vi "點檢_VI_畫十字線.vi"(8 "error in (no error)":errorcluster, 11 "Refnum in":T1) -> (0 "error out":errorcluster, 2 "中心點":cluster{sgl, sgl}, 3 "Refnum out":T1)   [LabVIEW 2015]
uses:
  <vilib>/vision/Image Controls.llb/IMAQ Image.ctl
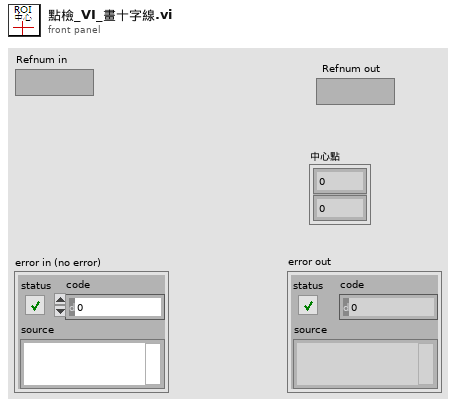
[diagram p1: front panel]
types:
  T1 = typedef "IMAQ Image.ctl" = refnum<image>
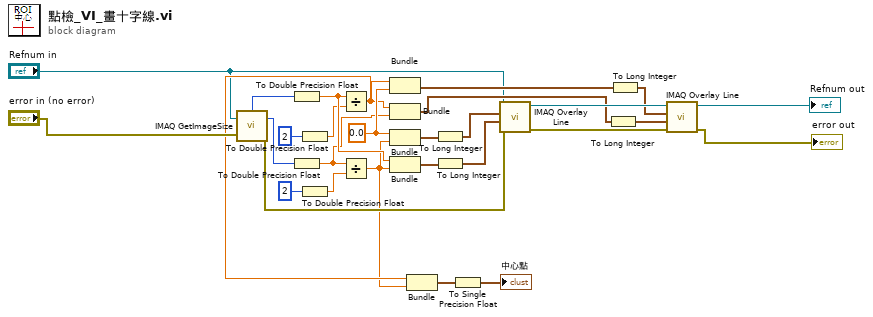
[diagram p0: block diagram]
diagram:
  w20 = 0.0
  n1 = call "IMAQ GetImageSize"("Image"="Refnum in", "error in (no error)"="error in (no error)") -> ("Y Resolution"=w24:i32, "X Resolution"=w3:i32, "error out"=w26:errorcluster)  [unwired: 2 in]
  n2 = To Double Precision Float(number=w3) -> (double precision float=w21:dbl)
  n3 = To Double Precision Float(number=w24) -> (double precision float=w19:dbl)
  n4 = To Double Precision Float(number=2 ("y")) -> (double precision float=w10:dbl)
  n5 = To Double Precision Float(number=2 ("y")) -> (double precision float=w9:dbl)
  n6 = Divide(x=w21, y=w10) -> (x/y=w7:dbl)
  n7 = Divide(x=w19, y=w9) -> (x/y=w6:dbl)
  n8 = Bundle(w7, w20) -> (w18:cluster{dbl, dbl})  [unwired: 1 in]
  n9 = Bundle(w7, w19) -> (w16:cluster{dbl, dbl})  [unwired: 1 in]
  n10 = Bundle(w20, w6) -> (w14:cluster{dbl, dbl})  [unwired: 1 in]
  n11 = Bundle(w21, w6) -> (w12:cluster{dbl, dbl})  [unwired: 1 in]
  n12 = Bundle(w7, w6) -> (w5:cluster{dbl, dbl})  [unwired: 1 in]
  n13 = To Long Integer(number=w14) -> (32bit integer=w13:cluster{i32, i32})
  n14 = To Long Integer(number=w12) -> (32bit integer=w11:cluster{i32, i32})
  n15 = To Single Precision Float(number=w5) -> (single precision float=→"中心點":cluster{sgl, sgl})
  n16 = call "IMAQ Overlay Line"("error in (no error)"=w26, "End Point"=w11, "Start Point"=w13, "Image"="Refnum in") -> ("error out"=w27:errorcluster, "Image Out"=w25:T1)  [unwired: 6 in]
  n17 = To Long Integer(number=w16) -> (32bit integer=w15:cluster{i32, i32})
  n18 = To Long Integer(number=w18) -> (32bit integer=w17:cluster{i32, i32})
  n19 = call "IMAQ Overlay Line"("error in (no error)"=w27, "End Point"=w15, "Start Point"=w17, "Image"=w25) -> ("error out"=→"error out":errorcluster, "Image Out"=→"Refnum out":T1)  [unwired: 6 in]
